vi "top score sort.vi"() -> ()   [LabVIEW 2014]
uses:
  <vilib>/Utility/miscctls.llb/LVRowAndColumnTypeDef.ctl
panel:
  out "Top 10 bar graph":dbl[](graph)
  out "Top 10 table":dbl[](array[numeric])
  out "sorted score":dbl[](array[numeric])
  out "sorted ID":i32[](array[numeric])
  out "Table":string[][](table)
  out "Score":dbl[](array[numeric])
  in  "Minimum":dbl=20.0
  in  "Maximum":dbl=80.0
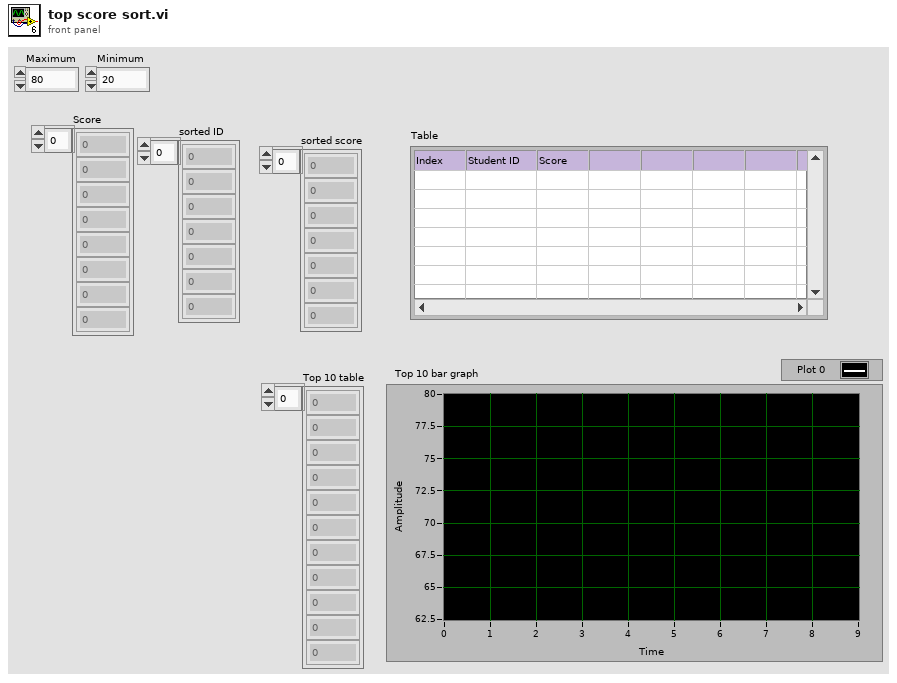
[diagram p1: front panel]
types:
  T1 = typedef "LVRowAndColumnTypeDef.ctl" = cluster{"Row":i32, "Column":i32}
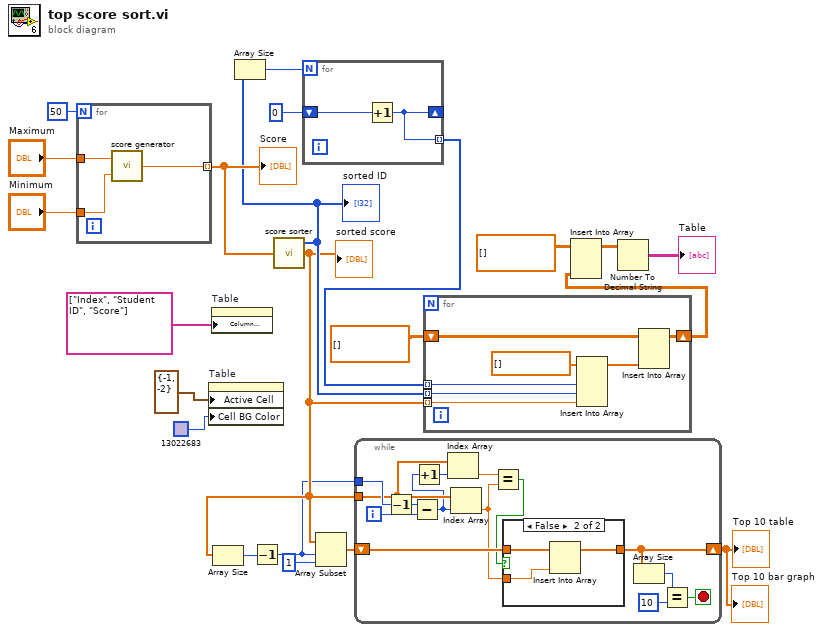
[diagram p0: block diagram]
diagram:
  n1 = for {
    N: 50 -> [_]
    tunnel: "Maximum" -> [w25]
    tunnel: "Minimum" -> [w24]
    tunnel: [w23] -> w18 mode=indexing
    n2 = call "score generator.vi"("Minimum"=w24, "Maximum"=w25) -> ("score"=w23:dbl)
  }
  "Score" <- w18
  n3 = property on="Table" class="Tbl (strict)"("Active Cell"=T1 {"Row"=-1, "Column"=-2} ("Active Cell:Active Cell"), "Cell BG Color"=u32 13022683 ("Color Box")) -> ()  [unwired: 2 in, 2 out]
  n4 = property on="Table" class="Tbl (strict)"("Column Headers[]"=string[] ["Index", "Student ID", "Score"] ("Row Header Strings[]")) -> ()  [unwired: 2 in, 2 out]
  n5 = call "score sorter.vi"("Score"=w18) -> ("sorted ID"=w12:i32[], "sorted score"=w4:dbl[])  [unwired: 1 out]
  "sorted ID" <- w12
  "sorted score" <- w4
  n6 = Array Size(array=w4) -> (size(s)=w3:i32)
  n7 = Array Size(array=w12) -> (size(s)=w17:i32)
  n8 = Decrement(x=w3) -> (x-1=w2:i32)
  n9 = for {
    N: w17 -> [_]
    shift-right: [w26] -> _
    shift-left: 0 -> [w27]
    tunnel: [w26] -> w13 mode=indexing
    n10 = Increment(x=w27) -> (x+1=w26:i32)
  }
  n11 = Array Subset(array=w4, index=w2, length=1) -> (w6:dbl[])
  n12 = while {
    tunnel: w4 -> [w33]
    shift-right: [w39] -> w1
    shift-left: w6 -> [w40]
    tunnel: w2 -> [w35]
    i -> [w41]
    stop <- w37 stop-if-true
    n13 = Decrement(x=w35) -> (x-1=w34:i32)
    n14 = Subtract(x=w34, y=w41) -> (x-y=w28:i32)
    n15 = Increment(x=w28) -> (x+1=w29:i32)
    n16 = Index Array(array=w33, index=w29) -> (element=w32:dbl)
    n17 = Index Array(array=w33, index=w28) -> (element=w31:dbl)
    n18 = Equal?(x=w32, y=w31) -> (x = y?=w30:bool)
    n19 = case shown="False" w30 {
      tunnel: w31 -> [_ w45]
      tunnel: [w42 w44] -> w39
      tunnel: w40 -> [w42 w43]
      frame True {
      }
      frame False {
        n20 = Insert Into Array(array=w43, new element=w45) -> (w44:dbl[])  [unwired: 1 in]
      }
    }
    n21 = Array Size(array=w39) -> (size(s)=w38:i32)
    n22 = Equal?(x=w38, y=10) -> (x = y?=w37:bool)
  }
  "Top 10 table" <- w1
  "Top 10 bar graph" <- w1
  n23 = for {
    tunnel: w13 -> [w52] mode=indexing
    tunnel: w12 -> [w51] mode=indexing
    tunnel: w4 -> [w50] mode=indexing
    shift-right: [w46] -> w7
    shift-left: dbl[][] [] -> [w47]
    n24 = Insert Into Array(array=dbl[] [], new element #1=w52, new element #2=w51, new element #3=w50) -> (w49:dbl[])  [unwired: 1 in]
    n25 = Insert Into Array(array=w47, new element=w49) -> (w46:dbl[][])  [unwired: 2 in]
  }
  n26 = Insert Into Array(array=dbl[][] [], new element=w7) -> (w10:dbl[][])  [unwired: 2 in]
  n27 = Number To Decimal String(number=w10) -> (decimal integer string=→"Table":string[][])  [unwired: 1 in]
